vi "Acquisition_Interlock.vi"(0 "Local Control":bool) -> ()   [LabVIEW 2010]
uses:
  Controls/Trigger_Mode.ctl
  Globals/Dynamic_call_global.ph.vi
  Globals/Meas_global.vi
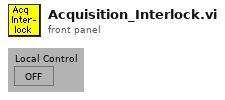
[diagram p1: front panel]
types:
  T1 = typedef "Trigger_Mode.ctl" = enum16{"Free Running", "Start on Trigger", "Trigger Every Block", "Trigger Every Sample"}
  T2 = typedef "Rendezvous RefNum" = refnum<k1>
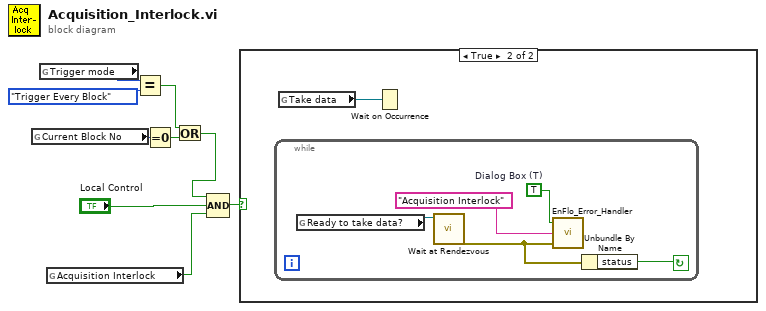
[diagram p0: block diagram]
diagram:
  n1 = global read "Meas_global.vi" "Current Block No"() -> (w6:i32)
  n2 = global read "Meas_global.vi" "Trigger mode"() -> (w4:T1)
  n3 = global read "Dynamic_call_global.ph.vi" "Acquisition Interlock"() -> (w9:bool)
  n4 = Equal?(x=w4, y=Trigger_Mode."Trigger Every Block" ("Trigger mode")) -> (x = y?=w2:bool)
  n5 = Equal To 0?(x=w6) -> (x = 0?=w5:bool)
  n6 = Or(x=w2, y=w5) -> (x .or. y?=w1:bool)
  n7 = Compound Arithmetic op=AND(w1, "Local Control", w9) -> (w8:bool)
  n8 = case shown="True" w8 {
    frame False {
    }
    frame True {
      n9 = while {
        stop <- w11 continue-if-true
        w13 = TRUE  # Dialog Box (T)
        n10 = global read "Dynamic_call_global.ph.vi" "Ready to take data?"() -> (w15:T2)
        n11 = call <vilib>:"Wait at Rendezvous.vi"("rendezvous"=w15) -> ("error out"=w12:errorcluster)  [unwired: 2 in, 4 out]
        n12 = call "EnFlo_Error_Handler.vi"("error in (no error)"=w12, "Error Type"="Acquisition Interlock", "Dialog Box (T)"=w13) -> ()  [unwired: 3 out]
        n13 = Unbundle By Name(w12) -> ("status"=w11:bool)
      }
      n14 = global read "Dynamic_call_global.ph.vi" "Take data"() -> (w10:refnum<k4>)
      n15 = Wait on Occurrence(2:w10) -> ()  [unwired: 3 out]
    }
  }
